vi "Tare Flow.vi"(7 "Unit ID (A)":string="A", 8 "error in":errorcluster, 11 "VISA Session In":refnum<visa-resource-name>="Alicat") -> (0 "error out":errorcluster, 3 "VISA Session Out":refnum<visa-resource-name>)   [LabVIEW 2016]
doc: "Performs a flow tare of an Alicat device."
uses:
  <vilib>/Instr/_visa.llb/VISA Flush IO Buffer Mask.ctl
panel:
  out "Data string returned":string
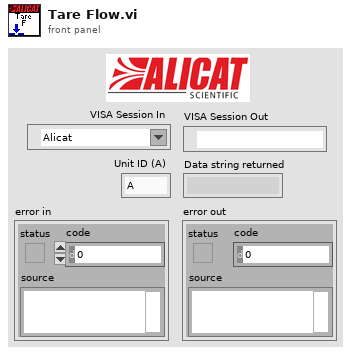
[diagram p1: front panel]
types:
  T1 = typedef "VISA Flush IO Buffer Mask.ctl" = u16
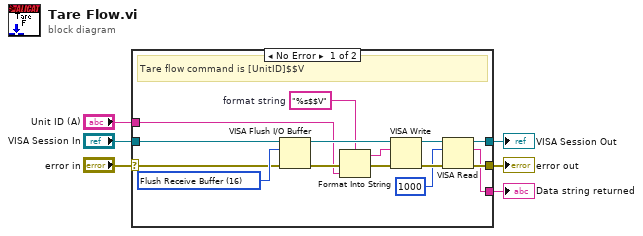
[diagram p0: block diagram]
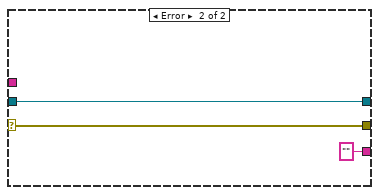
[diagram p2: hidden frame]
diagram:
  n1 = case shown="No Error" "error in" {
    selector: "error in" -> [w8 w23]
    tunnel: "VISA Session In" -> [w21 w24]
    tunnel: [w20 w24] -> w5
    tunnel: [w19 w23] -> w4
    tunnel: "Unit ID (A)" -> [w9 _]
    tunnel: [w7 "" ("read buffer")] -> w1
    frame No Error {
      w10 = T1 16 items=["Flush Receive Buffer"=16, "Write Transmit Buffer to Device"=32, "Flush Receive Buffer (No I/O)"=64, "Flush Transmit Buffer"=128] ("Mask")
      w15 = "%s$$V"  # format string
      # "Tare flow command is [UnitID]$$V"
      n2 = VISA Flush I/O Buffer(VISA resource name=w21, mask (16)=w10, error in (no error)=w8) -> (VISA resource name out=w17:refnum<visa-resource-name>, error out=w13:errorcluster)
      n3 = Format Into String(format string=w15, error in=w13, w9) -> (resulting string=w14:string, error out=w12:errorcluster)  [unwired: 1 in]
      n4 = VISA Write(VISA resource name=w17, write buffer=w14, error in (no error)=w12) -> (VISA resource name out=w16:refnum<visa-resource-name>, error out=w18:errorcluster)  [unwired: 1 out]
      n5 = VISA Read(VISA resource name=w16, byte count=u32 1000, error in (no error)=w18) -> (VISA resource name out=w20:refnum<visa-resource-name>, read buffer=w7:string, error out=w19:errorcluster)  [unwired: 1 out]
    }
    frame Error {
    }
  }
  "error out" <- w4
  "VISA Session Out" <- w5
  "Data string returned" <- w1
